vi "Shutdown.vi"(8 "error in (no error)":errorcluster, 11 "device data model in":refnum<class "Device Data Model.lvclass">) -> (0 "error out":errorcluster)   [LabVIEW 2018, in "SubVIs.lvlib" / "Device Data Model.lvclass"]
doc: "This VI is responsible for deleting the device data model."
uses:
  Device Data Model.lvclass
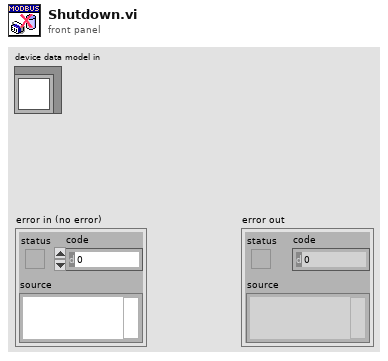
[diagram p1: front panel]
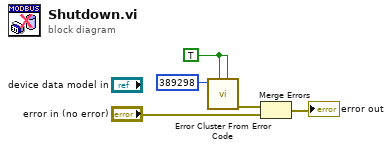
[diagram p0: block diagram]
diagram:
  w1 = TRUE ("show call chain? (False)")
  n1 = call "Error Cluster From Error Code.vi"("is warning? (False)"=w1, "show call chain? (False)"=w1, "error code (0)"=389298) -> ("error out"=w2:errorcluster)  [unwired: 6 in]
  n2 = Merge Errors(w2, "error in (no error)") -> (→"error out":errorcluster)
